vi "Get Ctrl Value.vi"(8 "error in (no error)":errorcluster, 11 "Text Field in":refnum<class "Text Field.lvclass">) -> (0 "error out":errorcluster, 2 "Ctrl Value":variant, 3 "Text Field out":refnum<class "Text Field.lvclass">)   [LabVIEW 2020]
uses:
  Text Field.lvclass
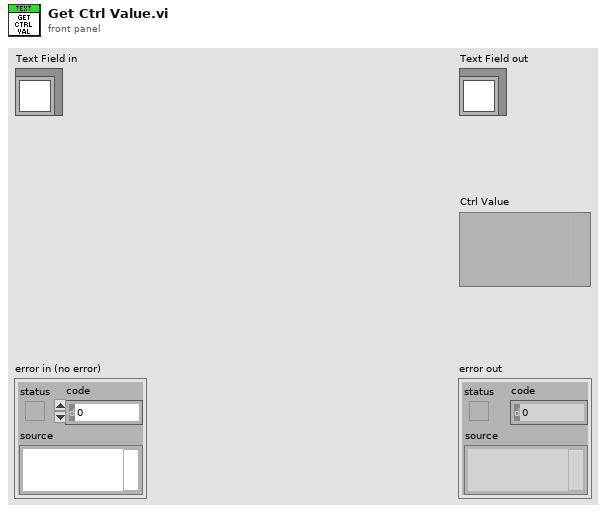
[diagram p1: front panel]
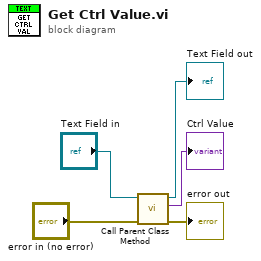
[diagram p0: block diagram]
diagram:
  n1 = call-parent "Call Parent Class Method"("error in (no error)"="error in (no error)", "Ctrl Refnum Column in"="Text Field in") -> ("error out"=→"error out":errorcluster, "Ctrl Value"=→"Ctrl Value":variant, "Ctrl Refnum Column out"=→"Text Field out":refnum<class "Text Field.lvclass">)  [unwired: 7 in]
